vi "VISA Initialize.vi"(8 "error in (no error)":errorcluster, 11 "Serial Settings":T1={"VISA"="", "Baud Rate"=9600, "Data Bits"=8, "Parity"=enum."None", "Stop Bits"=10, "Flow Control"=0} {"Flow Control" items=["None"=0, "XON/XOFF"=1, "RTS/CTS"=2, "DTR/DSR"=4]; "Stop Bits" items=["1.0"=10, "1.5"=15, "2.0"=20]; "Data Bits" min=5 max=8 step=1; "Baud Rate" items=["75"=75, "110"=110, "134"=134, "150"=150, "300"=300, "600"=600, "1200"=1200, "1800"=1800, "2400"=2400, "4800"=4800, "7200"=7200, "9600"=9600, "14400"=14400, "19200"=19200, "28800"=28800, "38400"=38400, "56000"=56000, "57600"=57600, "115200"=115200, "128000"=128000, "230400"=230400]}) -> (0 "error out":errorcluster, 3 "VISA Out":refnum<visa-resource-name>)   [LabVIEW 2014, in "VISA.lvlib"]
uses:
  VISA.lvlib
  <vilib>/Instr/_visa.llb/VISA Configure Serial Port (Instr).vi
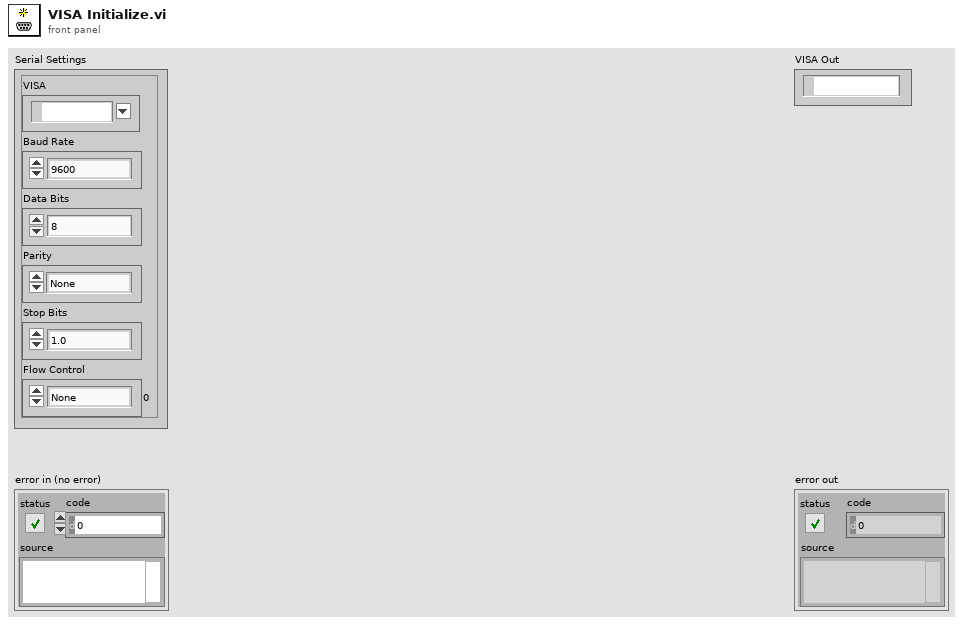
[diagram p1: front panel]
types:
  T1 = cluster{"VISA":refnum<visa-resource-name>, "Baud Rate":u32, "Data Bits":u16, "Parity":enum16{"None", "Odd", "Even", "Mark", "Space"}, "Stop Bits":u16, "Flow Control":u16}
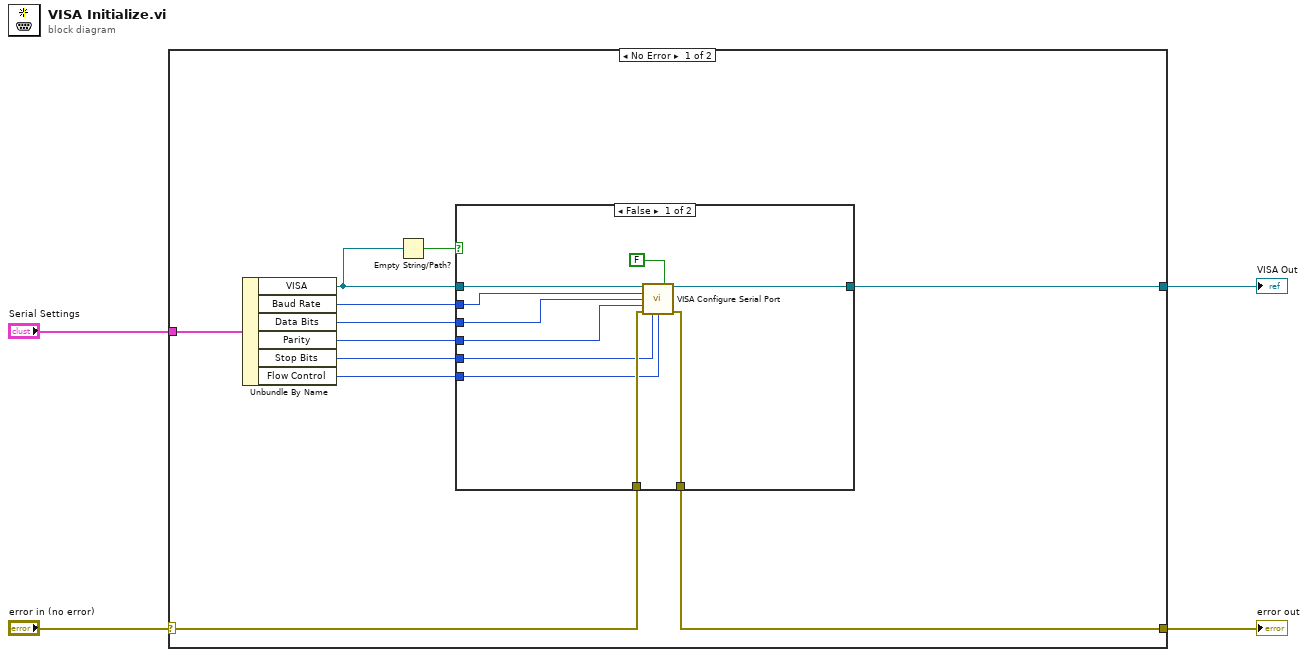
[diagram p0: block diagram]
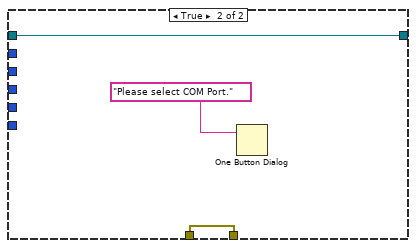
[diagram p2: hidden frame]
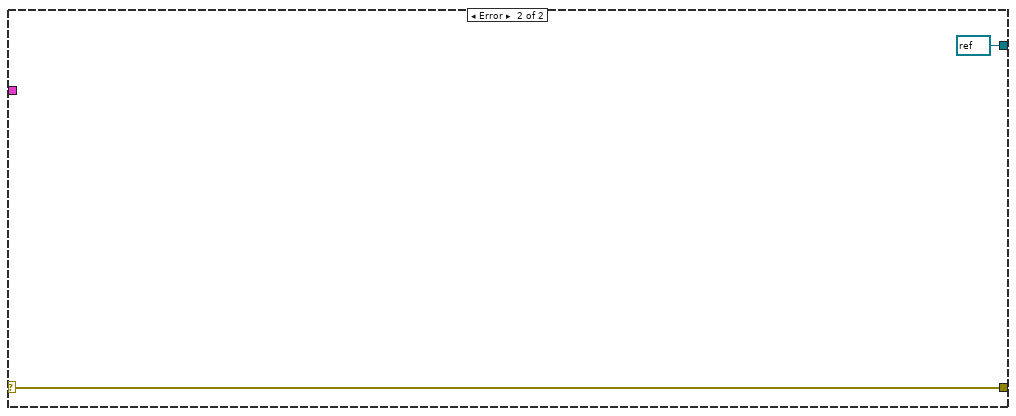
[diagram p3: hidden frame]
diagram:
  n1 = case shown="No Error" "error in (no error)" {
    selector: "error in (no error)" -> [w13 w30]
    tunnel: [w8 w30] -> w3
    tunnel: "Serial Settings" -> [w15 _]
    tunnel: [w7 refnum<visa-resource-name> refnum ("VISA resource name out")] -> w1
    frame No Error {
      n2 = Unbundle By Name(w15) -> ("VISA"=w5:refnum<visa-resource-name>, "Baud Rate"=w14:u32, "Data Bits"=w10:u16, "Parity"=w9:enum16{"None", "Odd", "Even", "Mark", "Space"}, "Stop Bits"=w12:u16, "Flow Control"=w11:u16)
      n3 = Empty String/Path?(string/path=w5) -> (empty?=w6:bool)
      n4 = case shown="False" w6 {
        tunnel: w14 -> [w25 _]
        tunnel: w13 -> [w24 w28]
        tunnel: w12 -> [w23 _]
        tunnel: w11 -> [w22 _]
        tunnel: w10 -> [w21 _]
        tunnel: w9 -> [w20 _]
        tunnel: [w19 w28] -> w8
        tunnel: [w18 w27] -> w7
        tunnel: w5 -> [w17 w27]
        frame False {
          n5 = call-poly "VISA Configure Serial Port"("VISA resource name"=w17, "Enable Termination\nChar (T)"=FALSE ("Enable Termination\nChar (T)"), "baud rate (9600)"=w25, "data bits (8)"=w21, "parity (0:none)"=w20, "error in (no error)"=w24, "stop bits (10: 1 bit)"=w23, "flow control (0:none)"=w22) -> ("VISA resource name out"=w18:refnum<visa-resource-name>, "error out"=w19:errorcluster)  [unwired: 6 in]
        }
        frame True {
          n6 = One Button Dialog(message="Please select COM Port.") -> ()  [unwired: 1 in, 1 out]
        }
      }
    }
    frame Error {
    }
  }
  "error out" <- w3
  "VISA Out" <- w1
